vi "Test_5110_3icon.vi"() -> ()   [LabVIEW 2021]
uses:
  ctrl/ini-rw.ctl
  ctrl/rw.ctl
  ctrl/5110_trigger.ctl
panel:
  in  "Tab Control":enum32{"User interface", "Config"}(tab)
  out "data 2":T1={"Waveform(s)"=[], "Actual Record Length"=1000, "Actual Sample Rate"=10000000.0, "Auto Triggered"=FALSE} {"Actual Sample Rate" format="%#.2p"}
  out "error out":errorcluster
  in  "stop":bool
  in  "cfg":T2={"visa"="PXI1Slot2", "Channel Name"="0", "Enforce Realtime"=TRUE, "Vertical Range"=4.0, "Min Sample Rate"=10000000.0, "Min Record Length"=3000, "Actual Record Length"=3000, "Actual Sample Rate"=10000000.0, "Timeout (s)"=5.0, "Vertical Offset"=0.0, "Probe Attenuation"=1.0, "Input Impedance"=0, "Maximum Input Frequency"=0.0, "Vertical Coupling"=1, "Trigger"={"Coupling"=1, "Trigger Slope"=0, "Trigger Level"=0.5, "Trigger Source"="0", "Trigger Delay"=0.0, "Reference Position"=50.0, "Trigger Modifier"=2, "Auto Triggered"=FALSE}} {"Trigger"."Trigger Modifier" items=["None"=1, "Auto Trigger"=2]; "Trigger"."Reference Position" format="%.1f"; "Trigger"."Trigger Delay" format="%#.4p"; "Trigger"."Trigger Level" format="%.2f"; "Trigger"."Trigger Slope" items=["Positive", "Negative"]; "Trigger"."Coupling" items=["AC"=0, "DC"=1, "HF Reject"=3, "LF Reject"=4, "AC Plus HF Reject"=1001]; "Vertical Coupling" items=["AC", "DC", "Ground"]; "Maximum Input Frequency" format="%.2f"; "Input Impedance" items=["1 mega ohm"=0, "50 ohms"=2]; "Probe Attenuation" format="%.1f"; "Vertical Offset" format="%.2p"; "Timeout (s)" format="%.2f"; "Actual Sample Rate" format="%#.2p"; "Min Sample Rate" step=1000000.0 format="%#.2p"; "Vertical Range" format="%.2f"}
  # "초음파 측정 PXI-5110"
  # "Vertical"
  # "Channel"
  # "Horizontal"
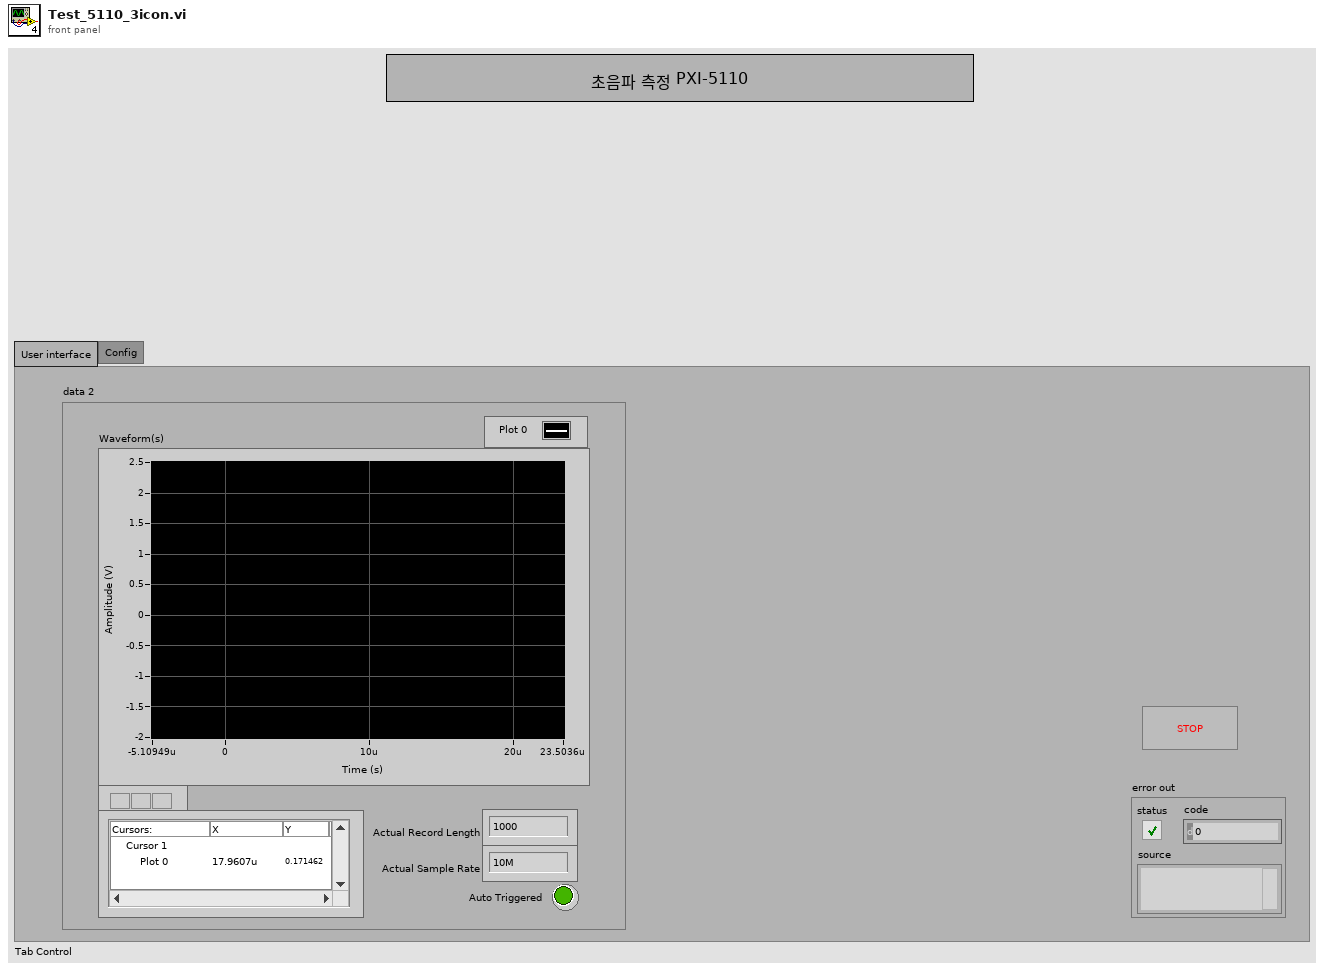
[diagram p1: front panel]
types:
  T1 = cluster{"Waveform(s)":cluster{"relativeInitialX":dbl, "xIncrement":dbl, "wfm":dbl[]}[], "Actual Record Length":i32, "Actual Sample Rate":dbl, "Auto Triggered":bool}
  T2 = typedef "5110_trigger.ctl" = cluster{"visa":refnum<k15>, "Channel Name":string, "Enforce Realtime":bool, "Vertical Range":dbl, "Min Sample Rate":dbl, "Min Record Length":i32, "Actual Record Length":i32, "Actual Sample Rate":dbl, "Timeout (s)":dbl, "Vertical Offset":dbl, "Probe Attenuation":dbl, "Input Impedance":u32, "Maximum Input Frequency":dbl, "Vertical Coupling":i32, "Trigger":cluster{"Coupling":u16, "Trigger Slope":i32, "Trigger Level":dbl, "Trigger Source":string, "Trigger Delay":dbl, "Reference Position":dbl, "Trigger Modifier":i32, "Auto Triggered":bool}}
  T3 = enum16{"init", "config", "trigger", "read", "close"}
  T4 = typedef "ini-rw.ctl" = enum16{"read", "write", "ini"}
  T5 = typedef "rw.ctl" = enum16{"read", "write"}
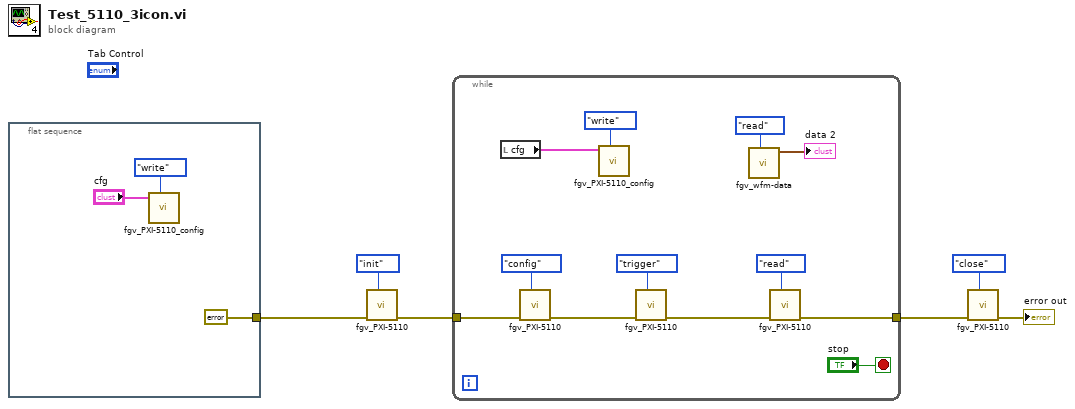
[diagram p0: block diagram]
diagram:
  n1 = flat-sequence {
    tunnel: [errorcluster {"status"=FALSE, "code"=0, "source"=""} ("error in")] -> w4
    frame #0 {
      n2 = call "fgv_PXI-5110_config.vi"("cmd"=ini-rw."write", "cfg"="cfg") -> ()  [unwired: 9 in, 1 out]
    }
  }
  n3 = call "fgv_PXI-5110.vi"("cmd"=T3."init", "error in"=w4) -> ("error out"=w5:errorcluster)  [unwired: 9 in]
  n4 = while {
    tunnel: w5 -> [w17]
    tunnel: [w20] -> w2
    stop <- "stop" stop-if-true
    n5 = local read "cfg"() -> (w10:T2)
    n6 = call "fgv_PXI-5110.vi"("cmd"=T3."config", "error in"=w17) -> ("error out"=w16:errorcluster)  [unwired: 9 in]
    n7 = call "fgv_PXI-5110_config.vi"("cmd"=ini-rw."write", "cfg"=w10) -> ()  [unwired: 9 in, 1 out]
    n8 = call "fgv_PXI-5110.vi"("cmd"=T3."trigger", "error in"=w16) -> ("error out"=w15:errorcluster)  [unwired: 9 in]
    n9 = call "fgv_wfm-data.vi"("cmd"=rw."read") -> ("wfm 2"=→"data 2":waveform(dbl))  [unwired: 10 in]
    n10 = call "fgv_PXI-5110.vi"("cmd"=T3."read", "error in"=w15) -> ("error out"=w20:errorcluster)  [unwired: 9 in]
  }
  n11 = call "fgv_PXI-5110.vi"("cmd"=T3."close", "error in"=w2) -> ("error out"=→"error out":errorcluster)  [unwired: 9 in]
